vi "Calculate Vertex Array.vi"(8 "error in (no error)":errorcluster, 9 "Coordinates System":enum16{"Cartesian", "Cylindrical", "Spherical"}(ring)=enum."Spherical", 10 "3D Mesh Datatype.lvclass in":refnum<class "3D Mesh Datatype.lvclass">, 11 "Plot Representation In":T1) -> (0 "error out":errorcluster, 1 "Dup Coordinates System":enum16{"Cartesian", "Cylindrical", "Spherical"}(ring)=enum."Spherical", 2 "3D Mesh Datatype.lvclass out":refnum<class "3D Mesh Datatype.lvclass">, 3 "Plot Representation Out":T1)   [LabVIEW 2020, in "3D Mesh Datatype.lvclass"]
uses:
  <vilib>/Math Plots/3D Math Plots/3D Mesh/3D Mesh Datatype/3D Mesh Datatype.lvclass
  <vilib>/Math Plots/3D Math Plots/3D Plot/3D Plot/Typedef/Plot Representation.ctl
  <vilib>/Math Plots/3D Math Plots/3D Plot/3D Plot/Typedef/Range Clusters.ctl
  <vilib>/Math Plots/3D Math Plots/3D Plot/3D Plot/Typedef/Mesh Data.ctl
  <vilib>/Math Plots/3D Math Plots/3D Mesh/3D Mesh Datatype/3D Mesh Datatype.lvclass/3D Mesh Datatype.ctl
  <vilib>/Math Plots/3D Math Plots/3D Plot/3D Plot Datatype/3D Plot Datatype.lvclass
  <vilib>/Math Plots/3D Math Plots/3D Plot/3D Plot/3D Plot.lvclass
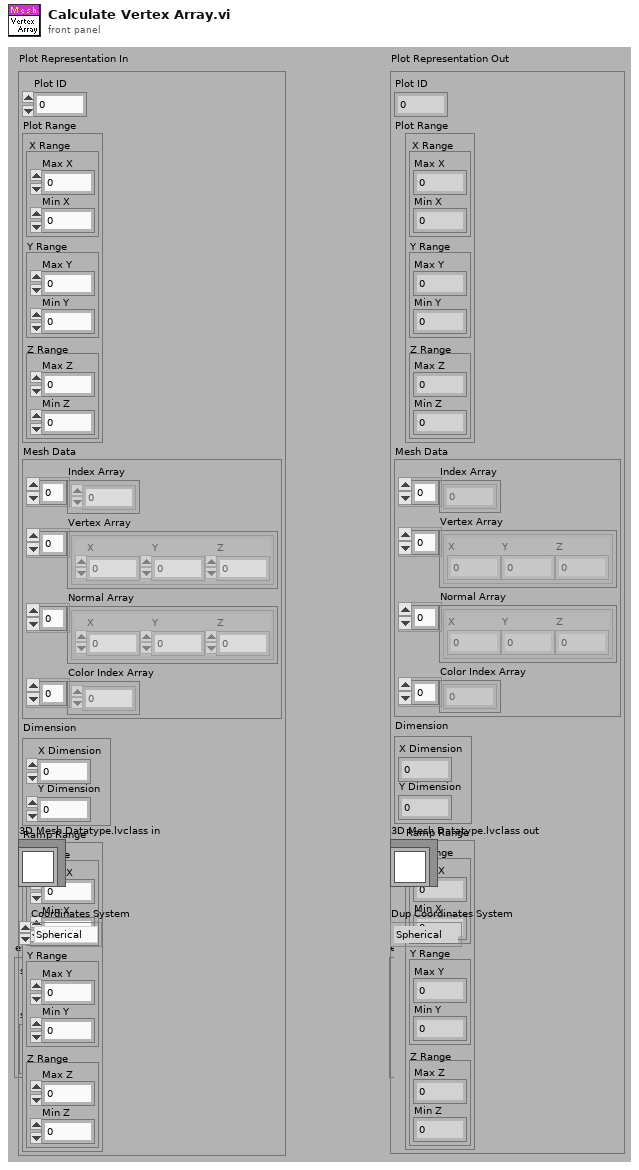
[diagram p1: front panel]
types:
  T1 = typedef "3D Plot.lvclass/Plot Representation.ctl" = cluster{"Plot ID":i32, "Plot Range":T2, "Mesh Data":T3, "Dimension":cluster{"X Dimension":i32, "Y Dimension":i32}, "Ramp Range":T2}
  T2 = typedef "3D Plot.lvclass/Range Clusters.ctl" = cluster{"X Range":cluster{"Max X":sgl, "Min X":sgl}, "Y Range":cluster{"Max Y":sgl, "Min Y":sgl}, "Z Range":cluster{"Max Z":sgl, "Min Z":sgl}}
  T3 = typedef "3D Plot.lvclass/Mesh Data.ctl" = cluster{"Index Array":u32[], "Vertex Array":cluster{"X":sgl, "Y":sgl, "Z":sgl}[], "Normal Array":cluster{"X":sgl, "Y":sgl, "Z":sgl}[], "Color Index Array":i32[]}
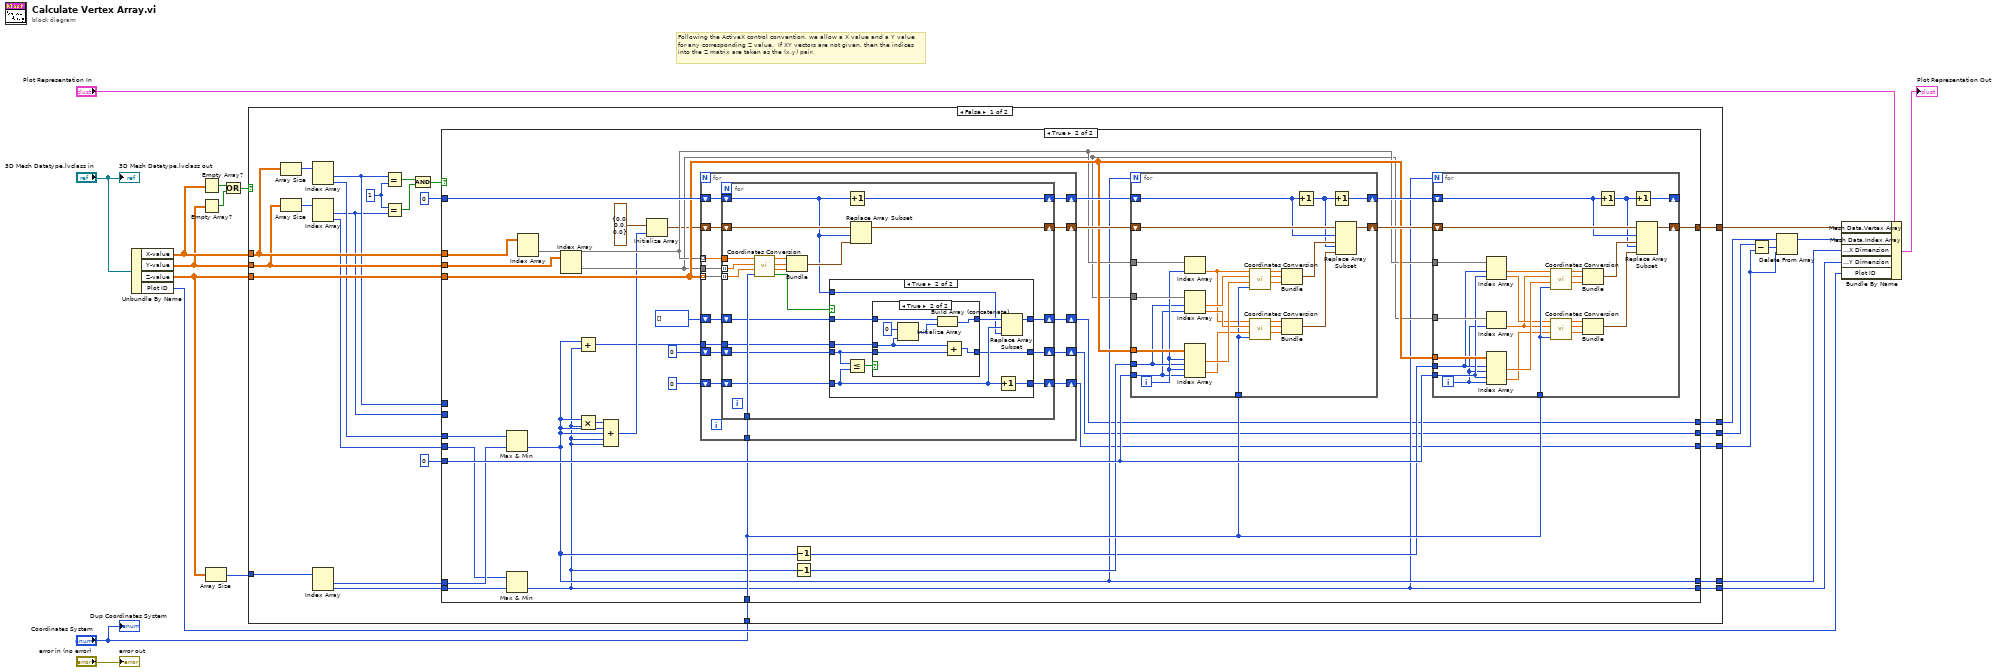
[diagram p0: block diagram]
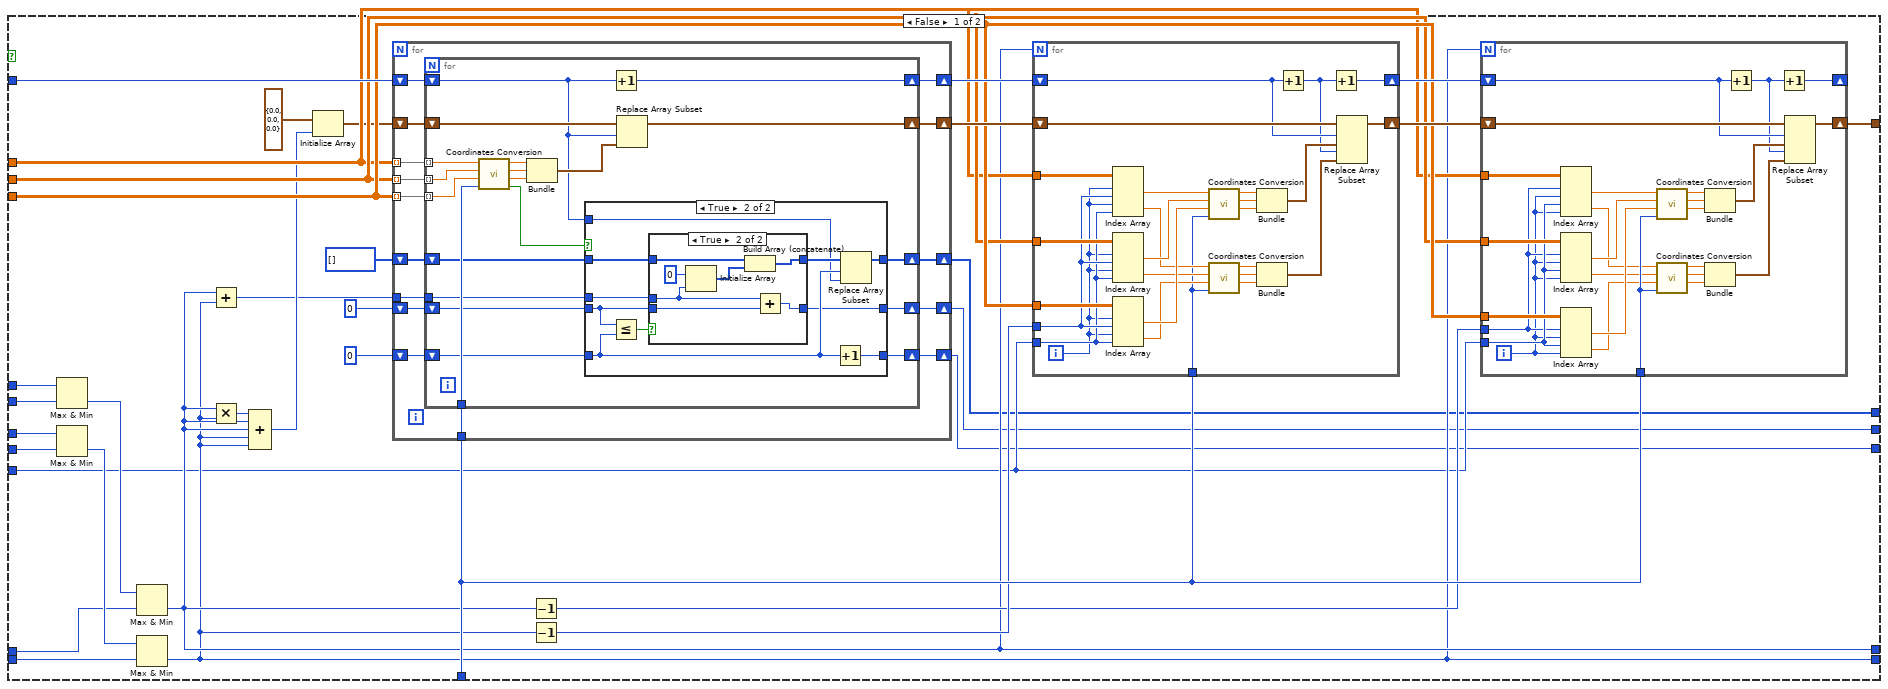
[diagram p2: hidden frame]
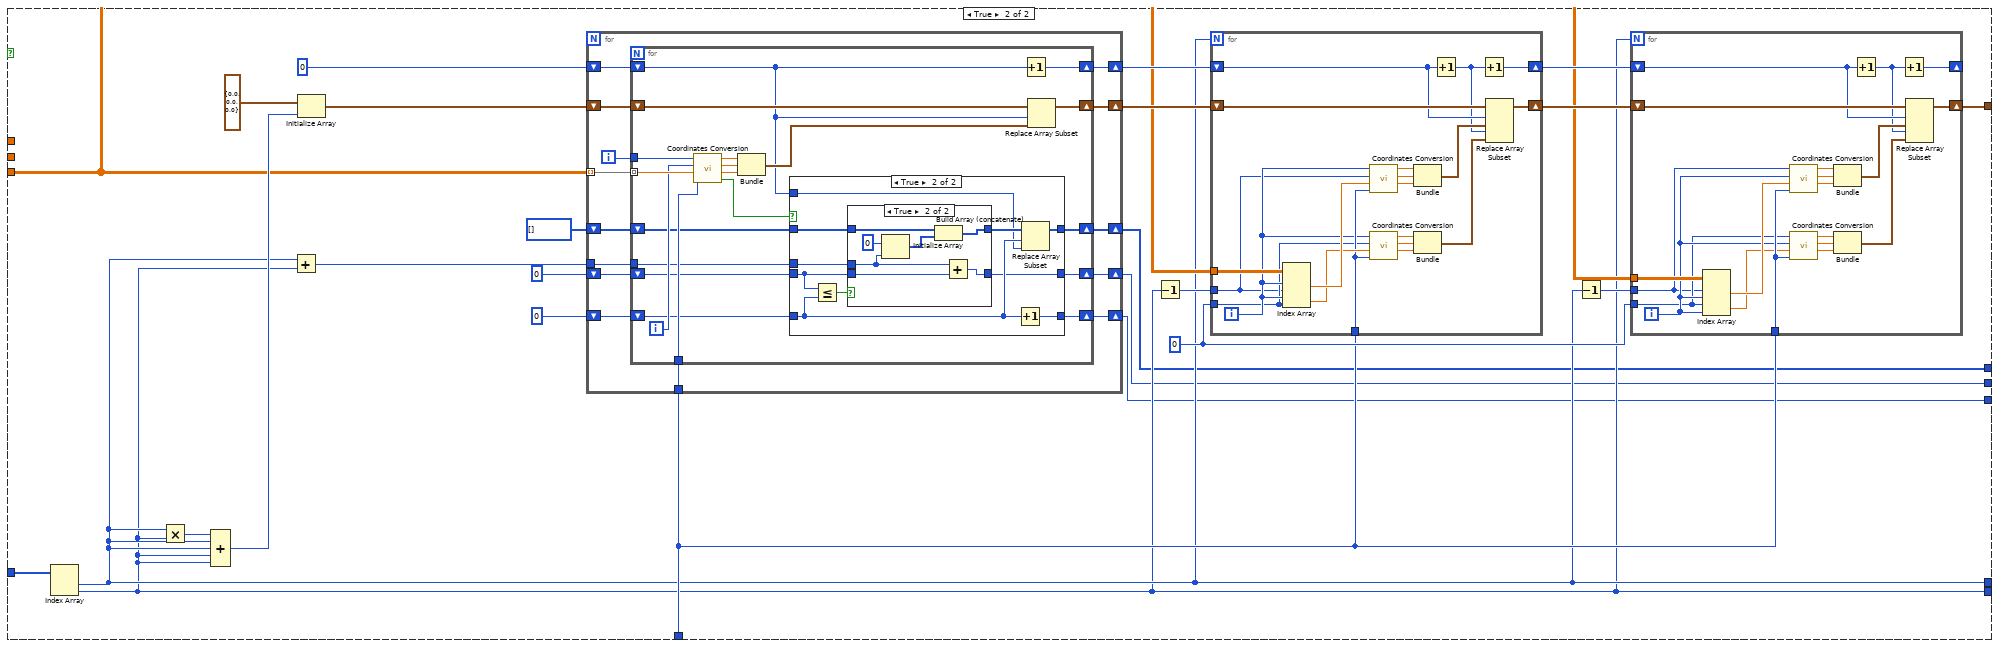
[diagram p7: hidden frame]
diagram:
  # "Following the ActiveX control convention, we allow a X value and a Y value for any corresponding Z value.  If XY vectors are not given, then the indices into the Z matrix are taken as the (x,y) pair."
  n1 = Unbundle By Name("3D Mesh Datatype.lvclass in") -> ("X-value"=w11:sgl[][], "Y-value"=w10:sgl[][], "Z-value"=w8:sgl[][], "Plot ID"=w16:i32)
  n2 = Empty Array?(array=w11) -> (empty?=w12:bool)
  n3 = Empty Array?(array=w10) -> (empty?=w13:bool)
  n4 = Array Size(array=w8) -> (size(s)=w7:i32[])
  n5 = Or(x=w12, y=w13) -> (x .or. y?=w9:bool)
  n6 = case shown="False" w9 {
    tunnel: "Coordinates System" -> [w29 w339]
    tunnel: [w46 w338] -> w17
    tunnel: w8 -> [w36 w340]
    tunnel: [w28 w334] -> w15
    tunnel: [w27 w333] -> w14
    tunnel: w11 -> [w37 _]
    tunnel: w10 -> [w34 _]
    tunnel: w7 -> [w43 w341]
    tunnel: [w24 w331] -> w3
    tunnel: [w23 w330] -> w2
    tunnel: [w22 w329] -> w1
    frame False {
      w40 = 1 ("x")
      n7 = Array Size(array=w37) -> (size(s)=w42:i32[])
      n8 = Array Size(array=w34) -> (size(s)=w41:i32[])
      n9 = Index Array(array=w42) -> (element #1=w26:i32, element #2=w33:i32)  [unwired: 2 in]
      n10 = Index Array(array=w41) -> (element #1=w25:i32, element #2=w31:i32)  [unwired: 2 in]
      n11 = Index Array(array=w43) -> (element #1=w32:i32, element #2=w30:i32)  [unwired: 2 in]
      n12 = Equal?(x=w26, y=w40) -> (x = y?=w39:bool)
      n13 = Equal?(x=w40, y=w25) -> (x = y?=w38:bool)
      n14 = And(x=w39, y=w38) -> (x .and. y?=w35:bool)
      n15 = case shown="True" w35 {
        tunnel: [w80 w210] -> w46
        tunnel: 0 -> [w50 w217]
        tunnel: 0 -> [w77 w216]
        tunnel: w34 -> [w73 w214]
        tunnel: w37 -> [w72 w215]
        tunnel: w36 -> [w74 w213]
        tunnel: w33 -> [w62 w206]
        tunnel: w32 -> [w57 w205]
        tunnel: w31 -> [w58 w204]
        tunnel: w30 -> [w59 w203]
        tunnel: w29 -> [w70 w202]
        tunnel: [w54 w195] -> w28
        tunnel: [w53 w194] -> w27
        tunnel: w26 -> [w64 _]
        tunnel: w25 -> [w63 _]
        tunnel: [w49 w192] -> w24
        tunnel: [w48 w191] -> w23
        tunnel: [w47 w190] -> w22
        frame False {
          n16 = Max & Min(x=w64, y=w63) -> (min(x,y)=w61:i32)  [unwired: 1 out]
          n17 = Max & Min(x=w62, y=w58) -> (min(x,y)=w60:i32)  [unwired: 1 out]
          n18 = Max & Min(x=w61, y=w57) -> (min(x,y)=w54:i32)  [unwired: 1 out]
          n19 = Max & Min(x=w60, y=w59) -> (min(x,y)=w53:i32)  [unwired: 1 out]
          n20 = Add(x=w54, y=w53) -> (x+y=w52:i32)
          n21 = Multiply(x=w54, y=w53) -> (x*y=w71:i32)
          n22 = Compound Arithmetic op=ADD(w71, w54, w54, w53, w53) -> (w65:i32)
          n23 = Initialize Array(cluster{"X":sgl, "Y":sgl, "Z":sgl} {"X"=0.0, "Y"=0.0, "Z"=0.0} ("3D Point"), w65) -> (w66:cluster{"X":sgl, "Y":sgl, "Z":sgl}[])
          n24 = for {
            shift-right: [w94] -> w78
            shift-left: w66 -> [w95]
            tunnel: w74 -> [w93] mode=indexing
            tunnel: w72 -> [w91] mode=indexing
            tunnel: w73 -> [w92] mode=indexing
            tunnel: w70 -> [w90]
            shift-right: [w88] -> w76
            shift-left: w77 -> [w89]
            shift-right: [w86] -> w49
            shift-left: u32[] [] -> [w87]
            shift-right: [w85] -> w48
            shift-left: 0 -> [w83]
            shift-right: [w84] -> w47
            shift-left: 0 -> [w82]
            tunnel: w52 -> [w81]
            n25 = for {
              tunnel: w93 -> [w111] mode=indexing
              shift-right: [w115] -> w94
              shift-left: w95 -> [w114]
              tunnel: w92 -> [w112] mode=indexing
              tunnel: w91 -> [w113] mode=indexing
              tunnel: w90 -> [w107]
              shift-right: [w105] -> w88
              shift-left: w89 -> [w104]
              shift-right: [w101] -> w86
              shift-left: w87 -> [w102]
              shift-right: [w100] -> w85
              shift-left: w83 -> [w98]
              shift-right: [w99] -> w84
              shift-left: w82 -> [w97]
              tunnel: w81 -> [w96]
              n26 = call <vilib>:"Coordinates Conversion.vi"("Coordinates System"=w107, "Z in"=w111, "Y in"=w112, "X in"=w113) -> ("NaN?"=w103:bool, "Z out"=w108:sgl, "Y out"=w109:sgl, "X out"=w110:sgl)  [unwired: 4 out]
              n27 = Bundle("X out"=w110, "Y out"=w109, "Z out"=w108) -> (w106:cluster{"X out":sgl, "Y out":sgl, "Z out":sgl})  [unwired: 1 out]
              n28 = case shown="True" w103 {
                tunnel: w102 -> [w118 w126]
                tunnel: [w118 w122] -> w101
                tunnel: w104 -> [_ w123]
                tunnel: w97 -> [w117 w124]
                tunnel: [w117 w128] -> w99
                tunnel: w98 -> [w116 w120]
                tunnel: [w116 w121] -> w100
                tunnel: w96 -> [_ w119]
                frame False {
                }
                frame True {
                  n29 = Less Or Equal?(x=w120, y=w124) -> (x <= y?=w127:bool)
                  n30 = case shown="True" w127 {
                    tunnel: w126 -> [w130 w137]
                    tunnel: [w130 w136] -> w125
                    tunnel: [w129 w132] -> w121
                    tunnel: w120 -> [w129 w133]
                    tunnel: w119 -> [_ w131]
                    frame False {
                    }
                    frame True {
                      n31 = Initialize Array(u32 0, w131) -> (w134:u32[])
                      n32 = Build Array (concatenate)(w137, w134) -> (w136:u32[])
                      n33 = Add(x=w131, y=w133) -> (x+y=w132:i32)
                    }
                  }
                  n34 = Increment(x=w124) -> (x+1=w128:i32)
                  n35 = Replace Array Subset(array=w125, new element=w123, index=w124) -> (w122:u32[])
                }
              }
              n36 = Increment(x=w104) -> (x+1=w105:i32)
              n37 = Replace Array Subset(array=w114, new element=w106, index=w104) -> (w115:cluster{"X":sgl, "Y":sgl, "Z":sgl}[])
            }
          }
          n38 = Decrement(x=w54) -> (x-1=w68:i32)
          n39 = Decrement(x=w53) -> (x-1=w69:i32)
          n40 = for {
            N: w54 -> [_]
            shift-right: [w159] -> w79
            shift-left: w78 -> [w160]
            tunnel: w74 -> [w161]
            tunnel: w72 -> [w163]
            tunnel: w73 -> [w162]
            tunnel: w69 -> [w158]
            tunnel: w50 -> [w157]
            tunnel: w70 -> [w143]
            shift-right: [w138] -> w75
            shift-left: w76 -> [w140]
            i -> [w156]
            n41 = Index Array(array=w163, index (row) #1=w156, index (col) #1=w158, index (row) #2=w156, index (col) #2=w157) -> (element #1=w155:sgl, element #2=w149:sgl)
            n42 = Index Array(array=w162, index (row) #1=w156, index (col) #1=w158, index (row) #2=w156, index (col) #2=w157) -> (element #1=w154:sgl, element #2=w148:sgl)
            n43 = Index Array(array=w161, index (row) #1=w156, index (col) #1=w158, index (row) #2=w156, index (col) #2=w157) -> (element #1=w153:sgl, element #2=w147:sgl)
            n44 = call <vilib>:"Coordinates Conversion.vi"("Coordinates System"=w143, "Z in"=w153, "Y in"=w154, "X in"=w155) -> ("Z out"=w150:sgl, "Y out"=w151:sgl, "X out"=w152:sgl)  [unwired: 5 out]
            n45 = call <vilib>:"Coordinates Conversion.vi"("Coordinates System"=w143, "Z in"=w147, "Y in"=w148, "X in"=w149) -> ("Z out"=w144:sgl, "Y out"=w145:sgl, "X out"=w146:sgl)  [unwired: 5 out]
            n46 = Bundle("X out"=w152, "Y out"=w151, "Z out"=w150) -> (w141:cluster{"X out":sgl, "Y out":sgl, "Z out":sgl})  [unwired: 1 out]
            n47 = Bundle("X out"=w146, "Y out"=w145, "Z out"=w144) -> (w142:cluster{"X out":sgl, "Y out":sgl, "Z out":sgl})  [unwired: 1 out]
            n48 = Increment(x=w140) -> (x+1=w139:i32)
            n49 = Increment(x=w139) -> (x+1=w138:i32)
            n50 = Replace Array Subset(array=w160, new element #1=w141, index #1=w140, new element #2=w142, index #2=w139) -> (w159:cluster{"X":sgl, "Y":sgl, "Z":sgl}[])
          }
          n51 = for {
            N: w53 -> [_]
            shift-right: [w185] -> w80
            shift-left: w79 -> [w186]
            tunnel: w74 -> [w187]
            tunnel: w72 -> [w189]
            tunnel: w73 -> [w188]
            tunnel: w68 -> [w183]
            tunnel: w50 -> [w184]
            tunnel: w70 -> [w182]
            shift-right: [w164] -> _
            shift-left: w75 -> [w166]
            i -> [w169]
            n52 = Index Array(array=w189, index (row) #1=w183, index (col) #1=w169, index (row) #2=w184, index (col) #2=w169) -> (element #1=w181:sgl, element #2=w175:sgl)
            n53 = Index Array(array=w188, index (row) #1=w183, index (col) #1=w169, index (row) #2=w184, index (col) #2=w169) -> (element #1=w180:sgl, element #2=w174:sgl)
            n54 = Index Array(array=w187, index (row) #1=w183, index (col) #1=w169, index (row) #2=w184, index (col) #2=w169) -> (element #1=w179:sgl, element #2=w173:sgl)
            n55 = call <vilib>:"Coordinates Conversion.vi"("Coordinates System"=w182, "Z in"=w179, "Y in"=w180, "X in"=w181) -> ("Z out"=w178:sgl, "Y out"=w177:sgl, "X out"=w176:sgl)  [unwired: 5 out]
            n56 = call <vilib>:"Coordinates Conversion.vi"("Coordinates System"=w182, "Z in"=w173, "Y in"=w174, "X in"=w175) -> ("Z out"=w170:sgl, "Y out"=w171:sgl, "X out"=w172:sgl)  [unwired: 5 out]
            n57 = Bundle("X out"=w176, "Y out"=w177, "Z out"=w178) -> (w167:cluster{"X out":sgl, "Y out":sgl, "Z out":sgl})  [unwired: 1 out]
            n58 = Bundle("X out"=w172, "Y out"=w171, "Z out"=w170) -> (w168:cluster{"X out":sgl, "Y out":sgl, "Z out":sgl})  [unwired: 1 out]
            n59 = Increment(x=w166) -> (x+1=w165:i32)
            n60 = Increment(x=w165) -> (x+1=w164:i32)
            n61 = Replace Array Subset(array=w186, new element #1=w167, index #1=w166, new element #2=w168, index #2=w165) -> (w185:cluster{"X":sgl, "Y":sgl, "Z":sgl}[])
          }
        }
        frame True {
          n62 = Max & Min(x=w206, y=w205) -> (min(x,y)=w195:i32)  [unwired: 1 out]
          n63 = Max & Min(x=w204, y=w203) -> (min(x,y)=w194:i32)  [unwired: 1 out]
          n64 = Index Array(array=w215) -> (element=w212:sgl[])  [unwired: 2 in]
          n65 = Index Array(array=w214) -> (element=w211:sgl[])  [unwired: 2 in]
          n66 = Add(x=w195, y=w194) -> (x+y=w193:i32)
          n67 = Multiply(x=w195, y=w194) -> (x*y=w207:i32)
          n68 = Compound Arithmetic op=ADD(w207, w195, w195, w194, w194) -> (w199:i32)
          n69 = Initialize Array(cluster{"X":sgl, "Y":sgl, "Z":sgl} {"X"=0.0, "Y"=0.0, "Z"=0.0} ("3D Point"), w199) -> (w208:cluster{"X":sgl, "Y":sgl, "Z":sgl}[])
          n70 = for {
            shift-right: [w235] -> w220
            shift-left: w208 -> [w236]
            tunnel: w213 -> [w234] mode=indexing
            tunnel: w212 -> [w232] mode=indexing
            tunnel: w211 -> [w233]
            tunnel: w202 -> [w231]
            shift-right: [w229] -> w219
            shift-left: w216 -> [w230]
            shift-right: [w228] -> w192
            shift-left: u32[] [] -> [w225]
            shift-right: [w227] -> w191
            shift-left: 0 -> [w224]
            shift-right: [w226] -> w190
            shift-left: 0 -> [w223]
            tunnel: w193 -> [w222]
            n71 = for {
              tunnel: w234 -> [w252] mode=indexing
              shift-right: [w256] -> w235
              shift-left: w236 -> [w255]
              tunnel: w233 -> [w253] mode=indexing
              tunnel: w232 -> [w254]
              tunnel: w231 -> [w248]
              shift-right: [w246] -> w229
              shift-left: w230 -> [w242]
              shift-right: [w245] -> w228
              shift-left: w225 -> [w240]
              shift-right: [w244] -> w227
              shift-left: w224 -> [w239]
              shift-right: [w243] -> w226
              shift-left: w223 -> [w238]
              tunnel: w222 -> [w237]
              n72 = call <vilib>:"Coordinates Conversion.vi"("Coordinates System"=w248, "Z in"=w252, "Y in"=w253, "X in"=w254) -> ("NaN?"=w241:bool, "Z out"=w249:sgl, "Y out"=w250:sgl, "X out"=w251:sgl)  [unwired: 4 out]
              n73 = Bundle("X out"=w251, "Y out"=w250, "Z out"=w249) -> (w247:cluster{"X out":sgl, "Y out":sgl, "Z out":sgl})  [unwired: 1 out]
              n74 = case shown="True" w241 {
                tunnel: w240 -> [w259 w267]
                tunnel: [w259 w263] -> w245
                tunnel: w242 -> [_ w264]
                tunnel: w238 -> [w258 w265]
                tunnel: [w258 w269] -> w243
                tunnel: w239 -> [w257 w261]
                tunnel: [w257 w262] -> w244
                tunnel: w237 -> [_ w260]
                frame False {
                }
                frame True {
                  n75 = Less Or Equal?(x=w261, y=w265) -> (x <= y?=w268:bool)
                  n76 = case shown="True" w268 {
                    tunnel: w267 -> [w271 w278]
                    tunnel: [w271 w277] -> w266
                    tunnel: [w270 w273] -> w262
                    tunnel: w261 -> [w270 w274]
                    tunnel: w260 -> [_ w272]
                    frame False {
                    }
                    frame True {
                      n77 = Initialize Array(u32 0, w272) -> (w275:u32[])
                      n78 = Build Array (concatenate)(w278, w275) -> (w277:u32[])
                      n79 = Add(x=w272, y=w274) -> (x+y=w273:i32)
                    }
                  }
                  n80 = Increment(x=w265) -> (x+1=w269:i32)
                  n81 = Replace Array Subset(array=w266, new element=w264, index=w265) -> (w263:u32[])
                }
              }
              n82 = Increment(x=w242) -> (x+1=w246:i32)
              n83 = Replace Array Subset(array=w255, new element=w247, index=w242) -> (w256:cluster{"X":sgl, "Y":sgl, "Z":sgl}[])
            }
          }
          n84 = Decrement(x=w195) -> (x-1=w200:i32)
          n85 = Decrement(x=w194) -> (x-1=w201:i32)
          n86 = for {
            N: w195 -> [_]
            shift-right: [w299] -> w221
            shift-left: w220 -> [w300]
            tunnel: w213 -> [w301]
            tunnel: w212 -> [w303]
            tunnel: w211 -> [w302]
            tunnel: w201 -> [w280]
            tunnel: w217 -> [w279]
            tunnel: w202 -> [w287]
            shift-right: [w282] -> w218
            shift-left: w219 -> [w284]
            i -> [w298]
            n87 = Index Array(array=w303, index=w298) -> (element=w281:sgl)
            n88 = Index Array(array=w302, index #1=w280, index #2=w279) -> (element #1=w297:sgl, element #2=w292:sgl)
            n89 = Index Array(array=w301, index (row) #1=w298, index (col) #1=w280, index (row) #2=w298, index (col) #2=w279) -> (element #1=w296:sgl, element #2=w291:sgl)
            n90 = call <vilib>:"Coordinates Conversion.vi"("Coordinates System"=w287, "Z in"=w296, "Y in"=w297, "X in"=w281) -> ("Z out"=w293:sgl, "Y out"=w294:sgl, "X out"=w295:sgl)  [unwired: 5 out]
            n91 = call <vilib>:"Coordinates Conversion.vi"("Coordinates System"=w287, "Z in"=w291, "Y in"=w292, "X in"=w281) -> ("Z out"=w288:sgl, "Y out"=w289:sgl, "X out"=w290:sgl)  [unwired: 5 out]
            n92 = Bundle("X out"=w295, "Y out"=w294, "Z out"=w293) -> (w285:cluster{"X out":sgl, "Y out":sgl, "Z out":sgl})  [unwired: 1 out]
            n93 = Bundle("X out"=w290, "Y out"=w289, "Z out"=w288) -> (w286:cluster{"X out":sgl, "Y out":sgl, "Z out":sgl})  [unwired: 1 out]
            n94 = Increment(x=w284) -> (x+1=w283:i32)
            n95 = Increment(x=w283) -> (x+1=w282:i32)
            n96 = Replace Array Subset(array=w300, new element #1=w285, index #1=w284, new element #2=w286, index #2=w283) -> (w299:cluster{"X":sgl, "Y":sgl, "Z":sgl}[])
          }
          n97 = for {
            N: w194 -> [_]
            shift-right: [w324] -> w210
            shift-left: w221 -> [w325]
            tunnel: w213 -> [w326]
            tunnel: w212 -> [w328]
            tunnel: w211 -> [w327]
            tunnel: w200 -> [w322]
            tunnel: w217 -> [w323]
            tunnel: w202 -> [w321]
            shift-right: [w306] -> _
            shift-left: w218 -> [w308]
            i -> [w304]
            n98 = Index Array(array=w328, index #1=w322, index #2=w323) -> (element #1=w320:sgl, element #2=w315:sgl)
            n99 = Index Array(array=w327, index=w304) -> (element=w305:sgl)
            n100 = Index Array(array=w326, index (row) #1=w322, index (col) #1=w304, index (row) #2=w323, index (col) #2=w304) -> (element #1=w319:sgl, element #2=w314:sgl)
            n101 = call <vilib>:"Coordinates Conversion.vi"("Coordinates System"=w321, "Z in"=w319, "Y in"=w305, "X in"=w320) -> ("Z out"=w318:sgl, "Y out"=w317:sgl, "X out"=w316:sgl)  [unwired: 5 out]
            n102 = call <vilib>:"Coordinates Conversion.vi"("Coordinates System"=w321, "Z in"=w314, "Y in"=w305, "X in"=w315) -> ("Z out"=w311:sgl, "Y out"=w312:sgl, "X out"=w313:sgl)  [unwired: 5 out]
            n103 = Bundle("X out"=w316, "Y out"=w317, "Z out"=w318) -> (w309:cluster{"X out":sgl, "Y out":sgl, "Z out":sgl})  [unwired: 1 out]
            n104 = Bundle("X out"=w313, "Y out"=w312, "Z out"=w311) -> (w310:cluster{"X out":sgl, "Y out":sgl, "Z out":sgl})  [unwired: 1 out]
            n105 = Increment(x=w308) -> (x+1=w307:i32)
            n106 = Increment(x=w307) -> (x+1=w306:i32)
            n107 = Replace Array Subset(array=w325, new element #1=w309, index #1=w308, new element #2=w310, index #2=w307) -> (w324:cluster{"X":sgl, "Y":sgl, "Z":sgl}[])
          }
        }
      }
    }
    frame True {
      w352 = 0
      n108 = Index Array(array=w341) -> (element #1=w334:i32, element #2=w333:i32)  [unwired: 2 in]
      n109 = Multiply(x=w334, y=w333) -> (x*y=w343:i32)
      n110 = Compound Arithmetic op=ADD(w343, w334, w334, w333, w333) -> (w342:i32)
      n111 = Add(x=w334, y=w333) -> (x+y=w332:i32)
      n112 = Initialize Array(cluster{"X":sgl, "Y":sgl, "Z":sgl} {"X"=0.0, "Y"=0.0, "Z"=0.0} ("3D Point"), w342) -> (w348:cluster{"X":sgl, "Y":sgl, "Z":sgl}[])
      n113 = for {
        shift-right: [w366] -> w347
        shift-left: w348 -> [w367]
        tunnel: w340 -> [w365] mode=indexing
        tunnel: w339 -> [w364]
        shift-right: [w362] -> w345
        shift-left: 0 -> [w363]
        shift-right: [w358] -> w329
        shift-left: 0 -> [w356]
        shift-right: [w359] -> w330
        shift-left: 0 -> [w357]
        shift-right: [w360] -> w331
        shift-left: u32[] [] -> [w355]
        tunnel: w332 -> [w354]
        i -> [w361]
        n114 = for {
          tunnel: w365 -> [w384] mode=indexing
          shift-right: [w387] -> w366
          shift-left: w367 -> [w386]
          tunnel: w361 -> [w385]
          tunnel: w364 -> [w380]
          shift-right: [w378] -> w362
          shift-left: w363 -> [w375]
          shift-right: [w372] -> w358
          shift-left: w356 -> [w369]
          shift-right: [w373] -> w359
          shift-left: w357 -> [w370]
          shift-right: [w374] -> w360
          shift-left: w355 -> [w371]
          tunnel: w354 -> [w368]
          i -> [w377]
          n115 = call <vilib>:"Coordinates Conversion.vi"("Coordinates System"=w380, "Z in"=w384, "Y in"=w377, "X in"=w385) -> ("NaN?"=w376:bool, "Z out"=w381:sgl, "Y out"=w382:sgl, "X out"=w383:sgl)  [unwired: 4 out]
          n116 = Bundle("X out"=w383, "Y out"=w382, "Z out"=w381) -> (w379:cluster{"X out":sgl, "Y out":sgl, "Z out":sgl})  [unwired: 1 out]
          n117 = case shown="True" w376 {
            tunnel: w371 -> [w390 w398]
            tunnel: [w390 w394] -> w374
            tunnel: w375 -> [_ w395]
            tunnel: w369 -> [w389 w396]
            tunnel: [w389 w400] -> w372
            tunnel: w370 -> [w388 w392]
            tunnel: [w388 w393] -> w373
            tunnel: w368 -> [_ w391]
            frame False {
            }
            frame True {
              n118 = Less Or Equal?(x=w392, y=w396) -> (x <= y?=w399:bool)
              n119 = case shown="True" w399 {
                tunnel: w398 -> [w402 w409]
                tunnel: [w402 w408] -> w397
                tunnel: [w401 w404] -> w393
                tunnel: w392 -> [w401 w405]
                tunnel: w391 -> [_ w403]
                frame False {
                }
                frame True {
                  n120 = Initialize Array(u32 0, w403) -> (w406:u32[])
                  n121 = Build Array (concatenate)(w409, w406) -> (w408:u32[])
                  n122 = Add(x=w403, y=w405) -> (x+y=w404:i32)
                }
              }
              n123 = Increment(x=w396) -> (x+1=w400:i32)
              n124 = Replace Array Subset(array=w397, new element=w395, index=w396) -> (w394:u32[])
            }
          }
          n125 = Increment(x=w375) -> (x+1=w378:i32)
          n126 = Replace Array Subset(array=w386, new element=w379, index=w375) -> (w387:cluster{"X":sgl, "Y":sgl, "Z":sgl}[])
        }
      }
      n127 = Decrement(x=w333) -> (x-1=w351:i32)
      n128 = for {
        N: w334 -> [_]
        shift-right: [w427] -> w353
        shift-left: w347 -> [w428]
        tunnel: w340 -> [w429]
        tunnel: w351 -> [w410]
        tunnel: w352 -> [w411]
        tunnel: w339 -> [w418]
        shift-right: [w413] -> w344
        shift-left: w345 -> [w415]
        i -> [w412]
        n129 = Index Array(array=w429, index (row) #1=w412, index (col) #1=w410, index (row) #2=w412, index (col) #2=w411) -> (element #1=w426:sgl, element #2=w422:sgl)
        n130 = call <vilib>:"Coordinates Conversion.vi"("Coordinates System"=w418, "Z in"=w426, "Y in"=w410, "X in"=w412) -> ("Z out"=w423:sgl, "Y out"=w424:sgl, "X out"=w425:sgl)  [unwired: 5 out]
        n131 = call <vilib>:"Coordinates Conversion.vi"("Coordinates System"=w418, "Z in"=w422, "Y in"=w411, "X in"=w412) -> ("Z out"=w419:sgl, "Y out"=w420:sgl, "X out"=w421:sgl)  [unwired: 5 out]
        n132 = Bundle("X out"=w425, "Y out"=w424, "Z out"=w423) -> (w416:cluster{"X out":sgl, "Y out":sgl, "Z out":sgl})  [unwired: 1 out]
        n133 = Bundle("X out"=w421, "Y out"=w420, "Z out"=w419) -> (w417:cluster{"X out":sgl, "Y out":sgl, "Z out":sgl})  [unwired: 1 out]
        n134 = Increment(x=w415) -> (x+1=w414:i32)
        n135 = Increment(x=w414) -> (x+1=w413:i32)
        n136 = Replace Array Subset(array=w428, new element #1=w416, index #1=w415, new element #2=w417, index #2=w414) -> (w427:cluster{"X":sgl, "Y":sgl, "Z":sgl}[])
      }
      n137 = Decrement(x=w334) -> (x-1=w350:i32)
      n138 = for {
        N: w333 -> [_]
        shift-right: [w447] -> w338
        shift-left: w353 -> [w448]
        tunnel: w340 -> [w449]
        tunnel: w350 -> [w430]
        tunnel: w352 -> [w431]
        tunnel: w339 -> [w446]
        shift-right: [w433] -> _
        shift-left: w344 -> [w435]
        i -> [w432]
        n139 = Index Array(array=w449, index (row) #1=w430, index (col) #1=w432, index (row) #2=w431, index (col) #2=w432) -> (element #1=w445:sgl, element #2=w441:sgl)
        n140 = call <vilib>:"Coordinates Conversion.vi"("Coordinates System"=w446, "Z in"=w445, "Y in"=w432, "X in"=w430) -> ("Z out"=w444:sgl, "Y out"=w443:sgl, "X out"=w442:sgl)  [unwired: 5 out]
        n141 = call <vilib>:"Coordinates Conversion.vi"("Coordinates System"=w446, "Z in"=w441, "Y in"=w432, "X in"=w431) -> ("Z out"=w438:sgl, "Y out"=w439:sgl, "X out"=w440:sgl)  [unwired: 5 out]
        n142 = Bundle("X out"=w442, "Y out"=w443, "Z out"=w444) -> (w436:cluster{"X out":sgl, "Y out":sgl, "Z out":sgl})  [unwired: 1 out]
        n143 = Bundle("X out"=w440, "Y out"=w439, "Z out"=w438) -> (w437:cluster{"X out":sgl, "Y out":sgl, "Z out":sgl})  [unwired: 1 out]
        n144 = Increment(x=w435) -> (x+1=w434:i32)
        n145 = Increment(x=w434) -> (x+1=w433:i32)
        n146 = Replace Array Subset(array=w448, new element #1=w436, index #1=w435, new element #2=w437, index #2=w434) -> (w447:cluster{"X":sgl, "Y":sgl, "Z":sgl}[])
      }
    }
  }
  n147 = Subtract(x=w2, y=w1) -> (x-y=w5:i32)
  n148 = Delete From Array(array=w3, length=w5, index=w1) -> (array with subset deleted=w4:u32[])  [unwired: 1 out]
  n149 = Bundle By Name(cluster="Plot Representation In", "Mesh Data.Vertex Array"=w17, "Mesh Data.Index Array"=w4, "Dimension.X Dimension"=w15, "Dimension.Y Dimension"=w14, "Plot ID"=w16) -> (→"Plot Representation Out":T1)
  "error out" <- "error in (no error)"
  "3D Mesh Datatype.lvclass out" <- "3D Mesh Datatype.lvclass in"
  "Dup Coordinates System" <- "Coordinates System"
